vi "Set Timedloop Settings.vi"(8 "error in":errorcluster, 10 "Timed Loop Settings":T1={"Period(ms)"=2, "Priority"=100, "Processor"=-2}, 11 "Item Ref in":T2 format="%.0x") -> (0 "error out":errorcluster, 3 "Item Ref out":T2 format="%.0x")   [LabVIEW 2023, in "Vires VTD System Explorer.lvlib"]
uses:
  Vires VTD System Explorer.lvlib
  <vilib>/NI VeriStand/Custom Device API/Custom Device Item Ref.ctl
  Shared/Timedloop Settings.ctl
  Shared/Constants.vi
  <vilib>/NI VeriStand/Custom Device API/Set Item Property (Variant).vi
  Shared/Vires VTD Shared.lvlib
  <vilib>/NI VeriStand/Custom Device API/Custom Device API.lvlib
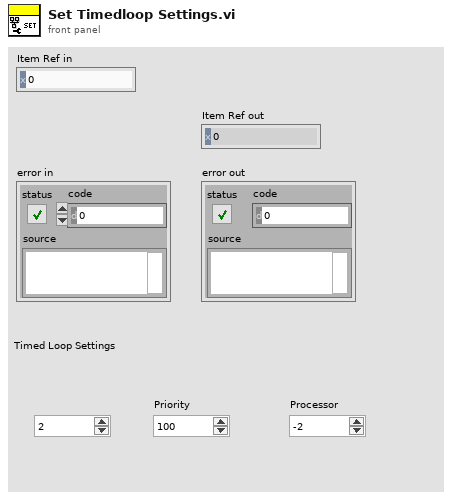
[diagram p1: front panel]
types:
  T1 = typedef "Vires VTD Shared.lvlib/Timedloop Settings.ctl" = cluster{"Period(ms)":i64, "Priority":i32, "Processor":i32}
  T2 = typedef "Custom Device API.lvlib/Custom Device Item Ref.ctl" = u64
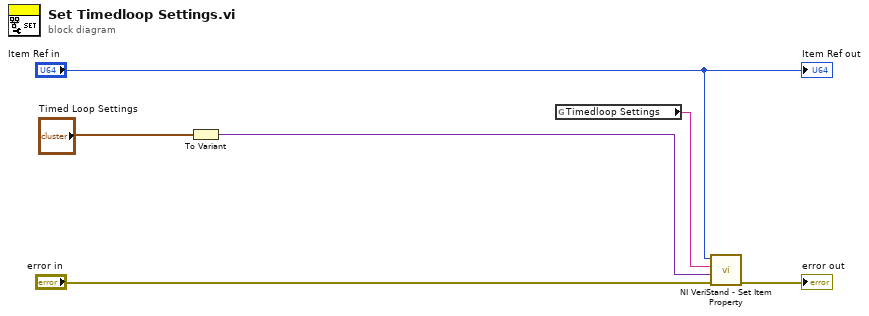
[diagram p0: block diagram]
diagram:
  n1 = To Variant(anything="Timed Loop Settings") -> (Variant=w5:variant)
  n2 = global read "Constants.vi" "Timedloop Settings"() -> (w6:string)
  n3 = call-poly <vilib>:"NI VeriStand - Set Item Property.vi"("error in (no error)"="error in", "Value"=w5, "Property Name"=w6, "Item Ref in"="Item Ref in") -> ("error out"=→"error out":errorcluster)  [unwired: 5 in, 2 out]
  "Item Ref out" <- "Item Ref in"
